vi "Draw Pixel.vi"(10 "Data":u16[](array[numeric])=[0, 0, 0, 0, 0, 0, 0, 0], 11 "Width":u16) -> ()   [LabVIEW 2019]
uses:
  <vilib>/rvi/Memory/Memory_Emulation/nirvimemoryFastEmulation.vi
  <vilib>/rvi/Memory/Memory_Emulation/nirvimemoryEmulation.vi
  <vilib>/rvi/Emulation/niFpgaEmulationIsFPGAContextNoSignature.vi
  <vilib>/rvi/DataTransferAndStorage/Container/Common/niFpgaContainerGetUniqueNameForEmu.vi
  <vilib>/rvi/Emulation/niFpgaProcessEmulError.vi
  <vilib>/rvi/Emulation/niFpgaSctlEmulationGetInTimedLoop.vi
  <vilib>/rvi/errors/nirviReportUnexpectedCaseInternalError (U32).vi
  <vilib>/rvi/DataTransferAndStorage/Container/XNode/niFpgaContainer.xnode
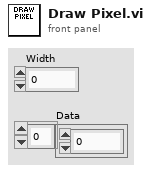
[diagram p1: front panel]
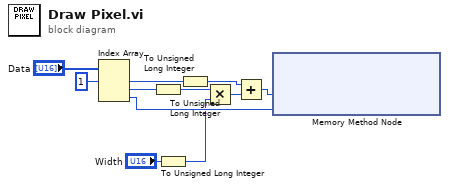
[diagram p0: block diagram]
diagram:
  n1 = Index Array(array="Data", index #1=1 ("index")) -> (element #1=w10:u16, element #2=w7:u16, element #3=w2:u16)  [unwired: 2 in]
  n2 = To Unsigned Long Integer(number=w7) -> (unsigned 32bit integer=w3:u32)
  n3 = To Unsigned Long Integer(number="Width") -> (unsigned 32bit integer=w1:u32)
  n4 = To Unsigned Long Integer(number=w10) -> (unsigned 32bit integer=w4:u32)
  n5 = Multiply(x=w3, y=w1) -> (x*y=w9:u32)
  n6 = Add(x=w4, y=w9) -> (x+y=w11:u32)
  n7 = xnode ("Memory Method Node")("Address"=w11, "Data"=w2) -> ()  [unwired: 1 in, 1 out]
